vi "HH_FileToImage.vi"(0 "Data In":u32[](array[numeric]), 1 "Reset":bool, 5 "Data Count":i32, 11 "Trace Bins":i32=25) -> (4 "Histograms":i32[][](array[numeric]), 6 "Total Photon Count":u64[](array[numeric]), 8 "Trigger Times":u64[](array[numeric]), 13 "Total Oveflow Count":u64, 14 "Num Records Total":i64, 15 "Traces":i32[][](array[numeric]))   [LabVIEW 2011]
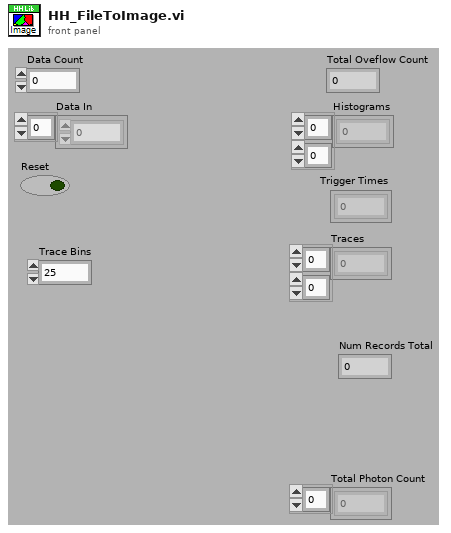
[diagram p1: front panel]
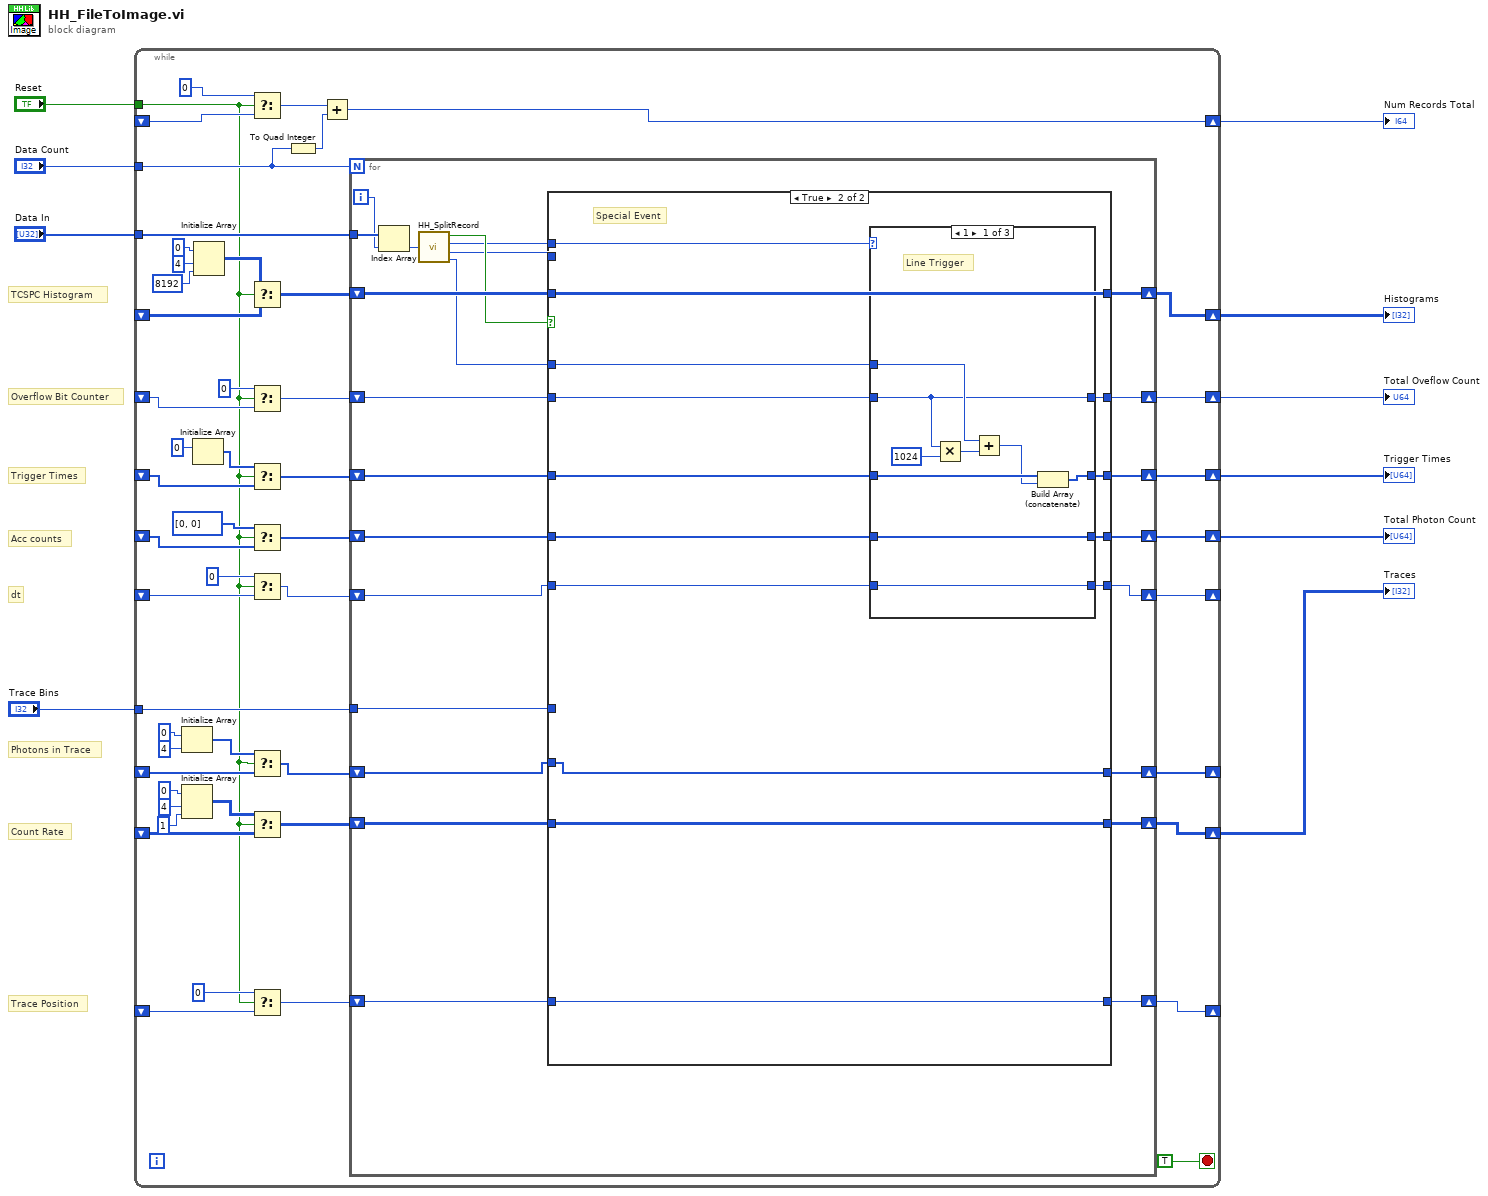
[diagram p0: block diagram]
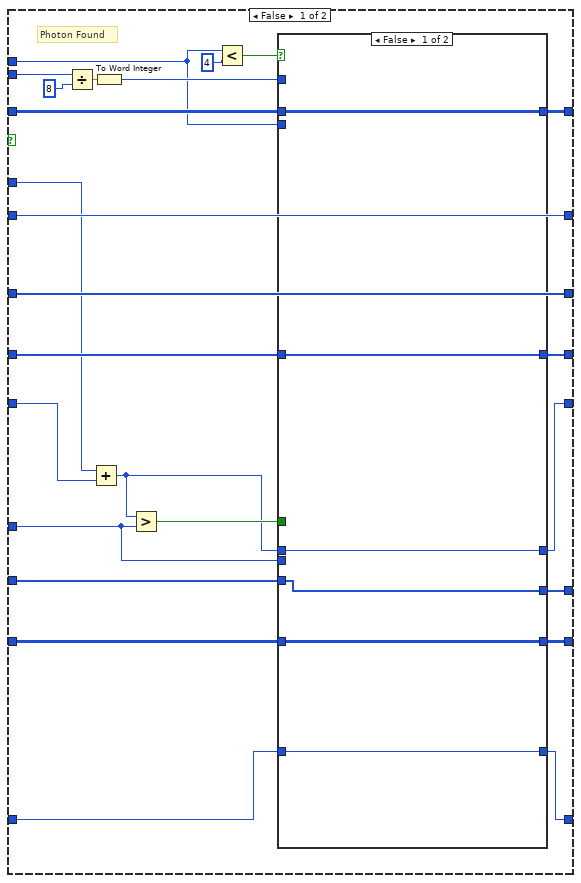
[diagram p2: hidden frame]
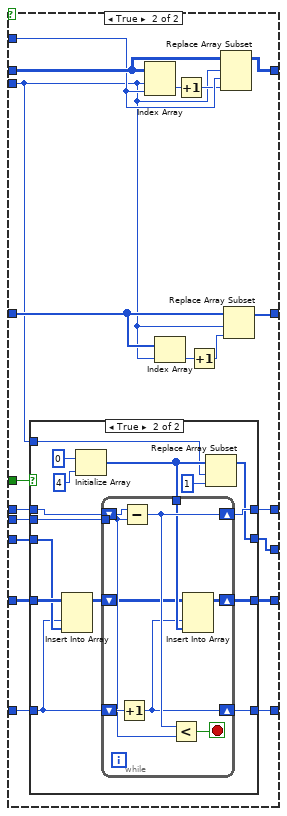
[diagram p3: hidden frame]
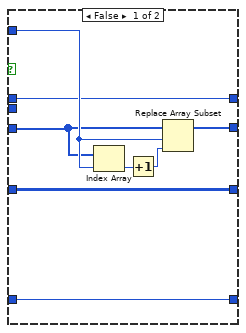
[diagram p4: hidden frame]
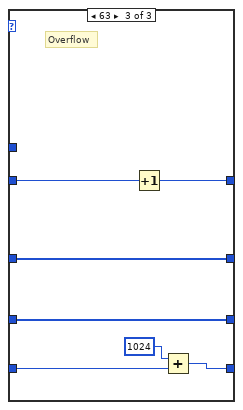
[diagram p6: hidden frame]
diagram:
  # "Photons in Trace"
  # "dt"
  # "Trace Position"
  # "Acc counts"
  # "Count Rate"
  # "Trigger Times"
  # "TCSPC Histogram"
  # "Overflow Bit Counter"
  n1 = while {
    tunnel: "Data In" -> [w59]
    shift-right: [w60] -> w10
    shift-left: _ -> [w55]
    tunnel: "Reset" -> [w12]
    shift-right: [w52] -> w3
    shift-left: _ -> [w51]
    shift-right: [w47] -> w7
    shift-left: _ -> [w46]
    shift-right: [w42] -> w6
    shift-left: _ -> [w41]
    tunnel: "Trace Bins" -> [w40]
    shift-right: [w37] -> _
    shift-left: _ -> [w36]
    tunnel: "Data Count" -> [w24]
    shift-right: [w32] -> w4
    shift-left: _ -> [w34]
    shift-right: [w26] -> w2
    shift-left: _ -> [w25]
    shift-right: [w20] -> _
    shift-left: _ -> [w19]
    shift-right: [w14] -> _
    shift-left: _ -> [w13]
    stop <- TRUE stop-if-true
    n2 = Initialize Array(0 ("element"), 4 ("dimension size")) -> (w17:i32[])
    n3 = Initialize Array(0 ("element"), 4 ("dimension size"), 1) -> (w44:i32[][])
    n4 = Initialize Array(u64 0 ("element")) -> (w49:u64[])  [unwired: 1 out]
    n5 = Initialize Array(0 ("element"), 4 ("dimension size"), 8192 ("dimension size")) -> (w56:i32[][])
    n6 = Select(t=i64 0 ("Data Count 2"), s=w12, f=w34) -> (s? t:f=w33:i64)
    n7 = Select(t=w56, s=w12, f=w55) -> (s? t:f=w57:i32[][])
    n8 = Select(t=u64 0, s=w12, f=w51) -> (s? t:f=w53:u64)
    n9 = Select(t=w49, s=w12, f=w46) -> (s? t:f=w48:u64[])
    n10 = Select(t=u64[] [0, 0] ("initialized array"), s=w12, f=w25) -> (s? t:f=w27:u64[])
    n11 = Select(t=u64 0, s=w12, f=w19) -> (s? t:f=w21:u64)
    n12 = Select(t=w17, s=w12, f=w13) -> (s? t:f=w15:i32[])
    n13 = Select(t=w44, s=w12, f=w41) -> (s? t:f=w43:i32[][])
    n14 = Select(t=0, s=w12, f=w36) -> (s? t:f=w38:i32)
    n15 = To Quad Integer(1:w24) -> (0:w23:i64)
    n16 = Add(x=w33, y=w23) -> (x+y=w32:i64)
    n17 = for {
      N: w24 -> [_]
      tunnel: w59 -> [w79]
      shift-right: [w84] -> w60
      shift-left: w57 -> [w85]
      shift-right: [w82] -> w52
      shift-left: w53 -> [w83]
      shift-right: [w80] -> w47
      shift-left: w48 -> [w81]
      shift-right: [w62] -> w42
      shift-left: w43 -> [w67]
      tunnel: w40 -> [w66]
      shift-right: [w63] -> w37
      shift-left: w38 -> [w68]
      shift-right: [w76] -> w26
      shift-left: w27 -> [w77]
      shift-right: [w64] -> w14
      shift-left: w15 -> [w65]
      shift-right: [w71] -> w20
      shift-left: w21 -> [w70]
      i -> [w78]
      n18 = Index Array(array=w79, index=w78) -> (element=w75:u32)
      n19 = call "HH_SplitRecord.vi"("Record in"=w75) -> ("Special"=w74:bool, "channel"=w73:i32, "time"=w72:i32, "nsync"=w69:u16)
      n20 = case shown="True" w74 {
        tunnel: w85 -> [w110 w180]
        tunnel: w73 -> [w93 w175]
        tunnel: [w109 w180] -> w84
        tunnel: w72 -> [w102 _]
        tunnel: w83 -> [w108 w182]
        tunnel: [w108 w181] -> w82
        tunnel: w81 -> [w107 w179]
        tunnel: [w107 w178] -> w80
        tunnel: w69 -> [w98 w169]
        tunnel: w77 -> [w104 w177]
        tunnel: [w103 w176] -> w76
        tunnel: w70 -> [w88 w174]
        tunnel: [w89 w173] -> w71
        tunnel: w67 -> [w96 w171]
        tunnel: w68 -> [w97 w172]
        tunnel: w66 -> [w86 _]
        tunnel: w65 -> [w95 w170]
        tunnel: [w90 w170] -> w64
        tunnel: [w92 w172] -> w63
        tunnel: [w91 w171] -> w62
        frame False {
          # "Photon Found"
          n21 = Divide(x=w102, y=8) -> (x/y=w101:dbl)
          n22 = Add(x=w98, y=w88) -> (x+y=w87:u64)
          n23 = To Word Integer(number=w101) -> (16bit integer=w99:i16)
          n24 = Greater?(x=w87, y=w86) -> (0:w94:bool)
          n25 = Less?(x=w93, y=4) -> (x < y?=w106:bool)
          n26 = case shown="False" w106 {
            tunnel: w110 -> [w116 w136]
            tunnel: [w116 w135] -> w109
            tunnel: w99 -> [_ w134]
            tunnel: w93 -> [_ w120]
            tunnel: w104 -> [w115 w129]
            tunnel: [w115 w128] -> w103
            tunnel: w97 -> [w114 w127]
            tunnel: w96 -> [w113 w126]
            tunnel: w95 -> [w112 w125]
            tunnel: w87 -> [w111 w119]
            tunnel: w94 -> [_ w124]
            tunnel: [w114 w123] -> w92
            tunnel: [w113 w122] -> w91
            tunnel: [w112 w121] -> w90
            tunnel: [w111 w118] -> w89
            tunnel: w86 -> [_ w117]
            frame False {
            }
            frame True {
              n27 = case shown="True" w124 {
                tunnel: w126 -> [w143 w159]
                tunnel: w127 -> [w144 w145]
                tunnel: [w143 w150] -> w122
                tunnel: [w144 w152] -> w123
                tunnel: w120 -> [w140 w146]
                tunnel: w125 -> [w138 w154]
                tunnel: [w139 w149] -> w121
                tunnel: w119 -> [w137 w155]
                tunnel: [w137 w156] -> w118
                tunnel: w117 -> [_ w153]
                frame False {
                  n28 = Index Array(array=w138, index=w140) -> (element=w141:i32)
                  n29 = Increment(x=w141) -> (x+1=w142:i32)
                  n30 = Replace Array Subset(array=w138, new element=w142, index=w140) -> (w139:i32[])
                }
                frame True {
                  n31 = Insert Into Array(array=w159, index (col)=w145, new element=w154) -> (w151:i32[][])  [unwired: 1 in]
                  n32 = Initialize Array(0, 4) -> (w148:i32[])
                  n33 = while {
                    tunnel: w153 -> [w164]
                    tunnel: w148 -> [w163]
                    shift-right: [w161] -> w150
                    shift-left: w151 -> [w162]
                    shift-right: [w160] -> w152
                    shift-left: w145 -> [w167]
                    shift-right: [w165] -> w156
                    shift-left: w155 -> [w168]
                    stop <- w166 stop-if-true
                    n34 = Increment(x=w167) -> (x+1=w160:i32)
                    n35 = Subtract(x=w168, y=w164) -> (x-y=w165:u64)
                    n36 = Less?(x=w165, y=w164) -> (x < y?=w166:bool)
                    n37 = Insert Into Array(array=w162, index (col)=w160, new element=w163) -> (w161:i32[][])  [unwired: 1 in]
                  }
                  n38 = Replace Array Subset(array=w148, new element=1, index=w146) -> (w149:i32[])
                }
              }
              n39 = Index Array(array=w136, index (row)=w120, index (col)=w134) -> (element=w133:i32)
              n40 = Index Array(array=w129, index=w120) -> (element=w131:u64)
              n41 = Increment(x=w133) -> (x+1=w132:i32)
              n42 = Increment(x=w131) -> (x+1=w130:u64)
              n43 = Replace Array Subset(array=w136, new element=w132, index (row)=w120, index (col)=w134) -> (w135:i32[][])
              n44 = Replace Array Subset(array=w129, new element=w130, index=w120) -> (w128:u64[])
            }
          }
        }
        frame True {
          # "Special Event"
          n45 = case shown="1" w175 {
            tunnel: w182 -> [w184 w195 w201]
            tunnel: [w184 w195 w200] -> w181
            tunnel: w179 -> [w191 w194 w202]
            tunnel: [w190 w194 w202] -> w178
            tunnel: w177 -> [w189 w193 w199]
            tunnel: [w189 w193 w199] -> w176
            tunnel: w174 -> [w187 w192 w198]
            tunnel: [w187 w192 w196] -> w173
            tunnel: w169 -> [w186 _ _]
            frame 1 {
              # "Line Trigger"
              n46 = Multiply(x=w184, y=1024) -> (x*y=w185:u64)
              n47 = Add(x=w186, y=w185) -> (x+y=w188:u64)
              n48 = Build Array (concatenate)(w191, w188) -> (w190:u64[])
            }
            frame Default {
            }
            frame 63 {
              # "Overflow"
              n49 = Increment(x=w201) -> (x+1=w200:u64)
              n50 = Add(x=1024, y=w198) -> (x+y=w196:u64)
            }
          }
        }
      }
    }
  }
  "Histograms" <- w10
  "Trigger Times" <- w7
  "Traces" <- w6
  "Num Records Total" <- w4
  "Total Oveflow Count" <- w3
  "Total Photon Count" <- w2
